vi "Phasor Compute Sum of Gates Plot.vi"(4 "SDV (s)":dbl=160.0, 6 "Gaussian IRF":bool, 8 "Error In":errorcluster, 10 "Phasor Parameters":T1={"Display Parameters"={"# Points"=0, "Ramp Type"=enum."Linear", "Type of Series"=enum."1-Exp Decays", "Min tau"=0.0, "Max tau"=0.0, "Include 0"=FALSE, "Include Infinity"=FALSE}, "Phasor Parameters"={"Harmonic Frequency"=0.0, "Use f* = 1/D Frequency"=FALSE, "Calibrated Phasor"=FALSE, "Calibration Lifetime"=1e-09, "Phasor Calculation"=enum."Direct Sum", "SEPL Type"=enum."UC", "# Gates"=1.0, "Square Gate Width"=1e-09, "Show Ticks"=FALSE}, "Decay & IRF Parameters"={"Lifetime"=0.0, "IRF Offset"=0.0, "IRF Period"=0.0, "Normalized Decays"=FALSE, "IRF Model"=enum."Dirac", "IRF Parameter 1"=0.0}, "Gate Parameters"={"First Gate Start"=0.0, "Use Gate Center"=FALSE, "Gate Width"=0.0, "Gate Step"=0.0, "# Gates"=0.0, "Gate Type"=enum."Square", "Edge Width"=0.0, "Top Slope"=0.0, "Reversed Sawtooth?"=FALSE, "Analytical Computation"=FALSE, "Integration"=enum."Item 0", "Tolerance"=1.0, "# Steps"=1.0, "Type of User-defined Function"=enum."Gate", "Use Gate Step"=FALSE}, "Detector Parameters"={"Frames/Image"=0, "Gates/Frame"=0, "Bits/Frame"=0, "Multiplicity"=0, "Incident Signal"=0.0, "Poisson Signal"=FALSE}} {"Detector Parameters"."Frames/Image" min=1; "Detector Parameters"."Multiplicity" min=0; "Detector Parameters"."Bits/Frame" min=1; "Detector Parameters"."Gates/Frame" min=1; "Gate Parameters"."# Steps" min=0.0; "Gate Parameters"."Tolerance" min=0.0; "Gate Parameters"."Top Slope" min=0.0; "Gate Parameters"."Edge Width" min=0.0; "Gate Parameters"."Gate Step" min=0.0; "Gate Parameters"."# Gates" min=0.0 step=1.0; "Gate Parameters"."Gate Width" min=0.0; "Decay & IRF Parameters"."Lifetime" min=0.0; "Decay & IRF Parameters"."IRF Period" min=0.0; "Phasor Parameters"."Square Gate Width" min=0.0; "Phasor Parameters"."# Gates" min=0.0; "Phasor Parameters"."Calibration Lifetime" min=0.0; "Phasor Parameters"."Harmonic Frequency" min=0.0; "Display Parameters"."Min tau" min=0.0; "Display Parameters"."Max tau" min=0.0; "Display Parameters"."# Points" min=1 step=1}, 11 "Sum of Gates Graph Refnum":refnum<vi>) -> (0 "Error Out":errorcluster, 3 "Sum of Gates Plot":cluster{"Array":dbl[], "Array":dbl[]})   [LabVIEW 2021, in "Phasor.lvlib"]
uses:
  Phasor.lvlib
  Arrays/Linear Ramp End Options.ctl
  Arrays/Arrays.lvlib
  Graphs/XY Graph/XY Graph Add-Ons.lvlib
  211736d7-2e51-4574-ab4f-80fa0041ca71.vi
  6eca1127-1b6c-4339-83be-8eda73648193.vi
  <vilib>/ErrorRing/Error Ring.xnode
  <vilib>/Utility/error.llb/Error Cluster From Error Code.vi
  Phasor Abort Parallel Computation.vi
  Graphs/XY Graph/XY Graph Add Single Plot with Name.vi
  Phasor SEPL Parameters.ctl
  Phasor Type of Series.ctl
  Phasor Explorer Display Parameters.ctl
  Phasor Explorer.lvlib
  Phasor Explorer Phasor Parameters.ctl
  Phasor Explorer Decay Parameters.ctl
  Phasor Explorer Gate Parameters.ctl
  Phasor Explorer Detector Parameters.ctl
  Phasor Calculation Type.ctl
  Phasor Gate Type.ctl
  Phasor SEPL Type.ctl
  Phasor IRF Model.ctl
  Phasor Type of User-defined Function.ctl
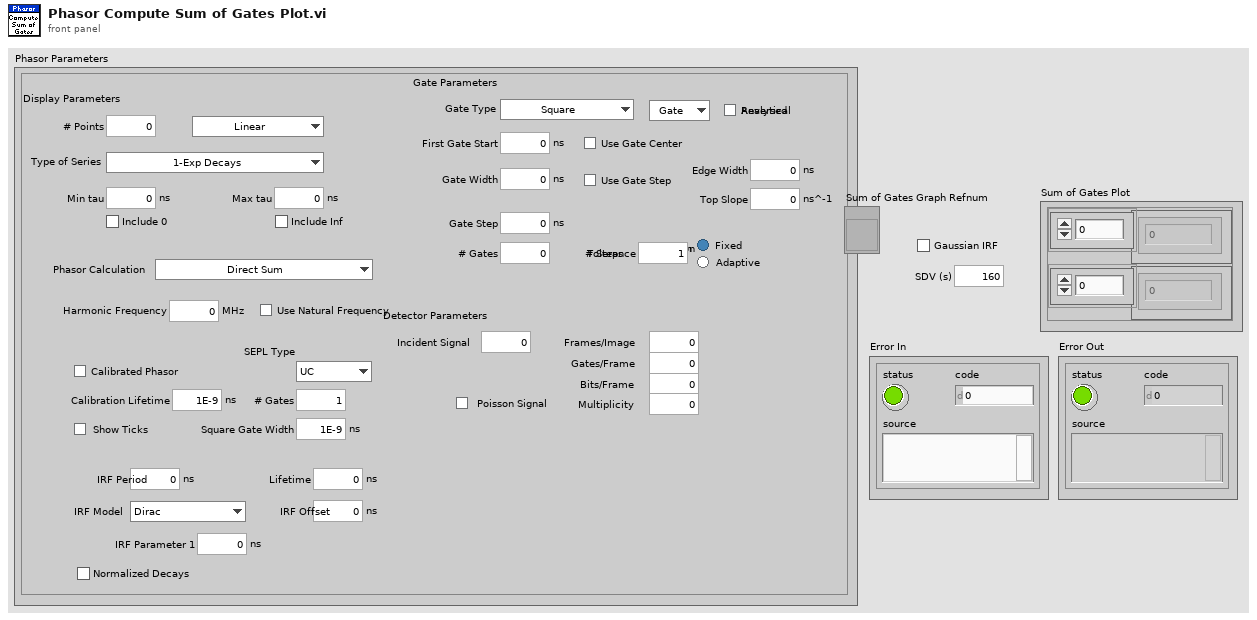
[diagram p1: front panel]
types:
  T1 = typedef "Phasor.lvlib/Phasor SEPL Parameters.ctl" = cluster{"Display Parameters":T2, "Phasor Parameters":T4, "Decay & IRF Parameters":T7, "Gate Parameters":T9, "Detector Parameters":T12}
  T2 = typedef "Phasor Explorer.lvlib/Phasor Explorer Display Parameters.ctl" = cluster{"# Points":i32, "Ramp Type":enum16{"Linear", "Logarithmic"}, "Type of Series":T3, "Min tau":dbl[unit], "Max tau":dbl[unit], "Include 0":bool, "Include Infinity":bool}
  T3 = typedef "Phasor.lvlib/Phasor Type of Series.ctl" = enum16{"1-Exp Decays", "Linear Combination of 1-Exp"}
  T4 = typedef "Phasor Explorer.lvlib/Phasor Explorer Phasor Parameters.ctl" = cluster{"Harmonic Frequency":dbl[unit], "Use f* = 1/D Frequency":bool, "Calibrated Phasor":bool, "Calibration Lifetime":dbl[unit], "Phasor Calculation":T5, "SEPL Type":T6, "# Gates":dbl, "Square Gate Width":dbl[unit], "Show Ticks":bool}
  T5 = typedef "Phasor.lvlib/Phasor Calculation Type.ctl" = enum16{"Direct Sum", "Analytical Formula"}
  T6 = typedef "Phasor.lvlib/Phasor SEPL Type.ctl" = enum16{"UC", "L_N", "L_N[W]", "L_X"}
  T7 = typedef "Phasor Explorer.lvlib/Phasor Explorer Decay Parameters.ctl" = cluster{"Lifetime":dbl[unit], "IRF Offset":dbl[unit], "IRF Period":dbl[unit], "Normalized Decays":bool, "IRF Model":T8, "IRF Parameter 1":dbl[unit]}
  T8 = typedef "Phasor.lvlib/Phasor IRF Model.ctl" = enum16{"Dirac", "Exponential"}
  T9 = typedef "Phasor Explorer.lvlib/Phasor Explorer Gate Parameters.ctl" = cluster{"First Gate Start":dbl[unit], "Use Gate Center":bool, "Gate Width":dbl[unit], "Gate Step":dbl[unit], "# Gates":dbl, "Gate Type":T10, "Edge Width":dbl[unit], "Top Slope":dbl[unit], "Reversed Sawtooth?":bool, "Analytical Computation":bool, "Integration":enum32{"Item 0", "Item 1"}, "Tolerance":dbl, "# Steps":dbl, "Type of User-defined Function":T11, "Use Gate Step":bool}
  T10 = typedef "Phasor.lvlib/Phasor Gate Type.ctl" = enum16{"Square", "Finite Edge Square", "Finite Edge, Tilted Top Square", "Triangle", "Sawtooth", "User-defined"}
  T11 = typedef "Phasor.lvlib/Phasor Type of User-defined Function.ctl" = enum16{"Gate", "IRF"}
  T12 = typedef "Phasor Explorer.lvlib/Phasor Explorer Detector Parameters.ctl" = cluster{"Frames/Image":i32, "Gates/Frame":i32, "Bits/Frame":i32, "Multiplicity":i32, "Incident Signal":dbl, "Poisson Signal":bool}
  T13 = typedef "Arrays.lvlib/Linear Ramp End Options.ctl" = enum16{"Include Min/Exclude Max", "Exclude Min/Include Max", "Include Both Ends", "Exclude Both Ends"}
  T14 = typedef "Phasor.lvlib/Phasor Gate Definitions.ctl" = cluster{"First Gate: t1":ext, "Gate Width: W":ext, "Gate Step: d":ext, "# Gates: G":ext, "Use Gate Center":bool, "Frames/Image: F":i32, "Gates/Frame: L":i32, "Bits/Frame: q":i32, "Multiplicity: p":i32, "Gate Type":T10, "Gate Edge s":ext, "Gate Top Slope":ext, "Reversed Sawtooth?":bool, "Computation":bool, "User-defined Gate":T15, "Tolerance":ext, "Integration":enum32{"Item 0", "Item 1"}, "# Steps":ext, "Type of User-defined Function":enum32{"Gate", "IRF"}}
  T15 = typedef "XY Graph Add-Ons.lvlib/XY Plot Data.ctl" = cluster{"X Array":dbl[], "Y Array":dbl[]}
  T16 = typedef "Phasor.lvlib/Phasor Decay Definiton.ctl" = cluster{"offset: t0":ext, "period: T":ext, "lifetime: tau":ext, "Incident Signal: I":ext, "Normalized Decays":bool, "IRF Model":T8, "IRF Parameter 1":ext, "Poisson Signal":bool}
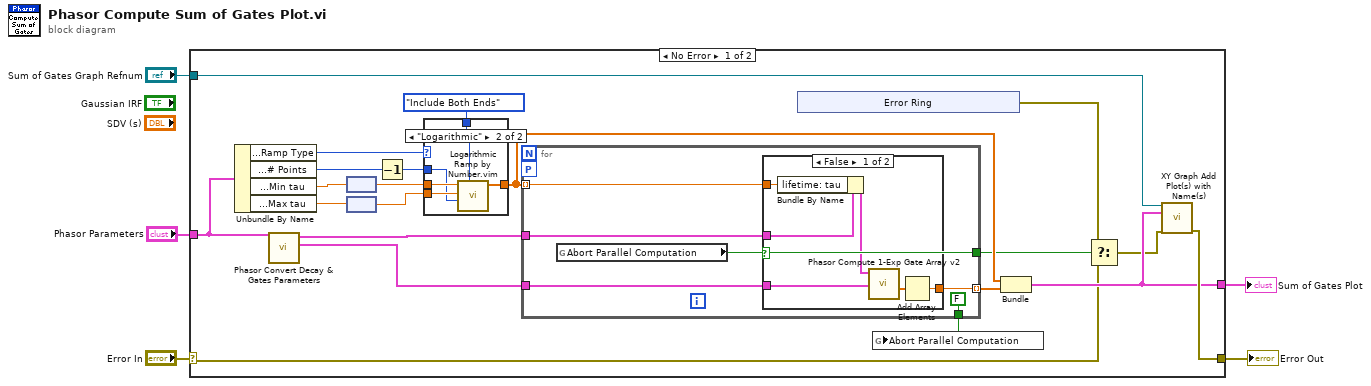
[diagram p0: block diagram]
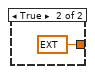
[diagram p2: hidden frame]
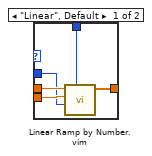
[diagram p3: hidden frame]
diagram:
  n1 = case shown="No Error" "Error In" {
    selector: "Error In" -> [w9 w54]
    tunnel: "Phasor Parameters" -> [w14 _]
    tunnel: "Sum of Gates Graph Refnum" -> [w22 _]
    tunnel: [w21 w54] -> w2
    tunnel: [w15 _] -> w1
    frame No Error {
      n2 = Unbundle By Name(w14) -> ("Display Parameters.Ramp Type"=w20:enum16{"Linear", "Logarithmic"}, "Display Parameters.# Points"=w17:i32, "Display Parameters.Min tau"=w25:dbl[unit], "Display Parameters.Max tau"=w26:dbl[unit])
      n3 = call "Phasor Convert Decay & Gates Parameters.vi"("Phasor Parameters"=w14) -> ("Gates Definitions"=w12:T14, "Decay Definition"=w13:T16)  [unwired: 9 in]
      n4 = node(w25) -> (w24:dbl)
      n5 = node(w26) -> (w23:dbl)
      n6 = Decrement(x=w17) -> (x-1=w18:i32)
      n7 = case shown="\"Logarithmic\"" w20 {
        tunnel: w24 -> [w48 w51]
        tunnel: w23 -> [w47 w50]
        tunnel: w18 -> [w46 w49]
        tunnel: [w45 w53] -> w11
        tunnel: Linear_Ramp_End_Options."Include Both Ends" ("Options") -> [w44 w52]
        frame "Linear", Default {
          n8 = call "Linear Ramp by Number.vim"("Options"=w44, "# Steps (1)"=w46, "End (1)"=w47, "Start (0)"=w48) -> ("Ramp"=w45:dbl[])  [unwired: 5 in, 2 out]
        }
        frame "Logarithmic" {
          n9 = call "Logarithmic Ramp by Number.vim"("Options"=w52, "# Steps (1)"=w49, "End (1)"=w50, "Start (1)"=w51) -> ("Ramp"=w53:dbl[])  [unwired: 6 in, 1 out]
        }
      }
      n10 = for {
        tunnel: w11 -> [w36] mode=indexing
        tunnel: w12 -> [w34]
        tunnel: w13 -> [w35]
        tunnel: [w33] -> w16 mode=indexing
        workers-P: _ -> [_]
        tunnel: [w32] -> w10
        tunnel: [FALSE ("Abort Parallel Computation")] -> w6
        n11 = global read "Phasor Abort Parallel Computation.vi" "Abort Parallel Computation"() -> (w32:bool)
        n12 = case shown="False" w32 {
          tunnel: w36 -> [w42 _]
          tunnel: w35 -> [w41 _]
          tunnel: w34 -> [w39 _]
          tunnel: [w37 ext nan ("Numeric Control")] -> w33
          frame False {
            n13 = Bundle By Name(cluster=w41, "lifetime: tau"=w42) -> (w40:T16)
            n14 = call "Phasor Compute 1-Exp Gate Array v2.vi"("Gates Definitions"=w39, "Decay Definition"=w40) -> ("Gate Image Array"=w38:ext[])  [unwired: 5 in, 4 out]
            n15 = Add Array Elements(numeric array=w38) -> (sum=w37:ext)
          }
          frame True {
          }
        }
      }
      n16 = xnode "Error Ring"() -> ("error out"=w7:errorcluster)
      n17 = global write "Phasor Abort Parallel Computation.vi" "Abort Parallel Computation"(w6) -> ()
      n18 = Bundle("Ramp"=w11, w16) -> (w15:cluster{"Ramp":dbl[], ext[]})  [unwired: 1 in]
      n19 = Select(t=w7, s=w10, f=w9) -> (s? t:f=w8:errorcluster)
      n20 = call-poly "XY Graph Add Plot(s) with Name(s).vi"("XYGraph Ref in"=w22, "Plot"=w15, "error in (no error)"=w8) -> ("error out"=w21:errorcluster)  [unwired: 9 in, 3 out]
    }
    frame Error {
    }
  }
  "Error Out" <- w2
  "Sum of Gates Plot" <- w1
